vi "Read Assert.vi"(7 "Assert Only? (F)":bool, 8 "error in (no error)":errorcluster, 10 "VI Call Chain":string[](array[string]), 11 "Assert Factory in":refnum<class "Assert Factory.lvclass">) -> (0 "error out":errorcluster, 2 "Assert":refnum<class "Assert.lvclass">, 3 "Assert Factory out":refnum<class "Assert Factory.lvclass">)   [LabVIEW 2009, in "Caraya.lvlib" / "Assert Factory.lvclass"]
doc: "Returns the Assert implementation being used for a specific VI."
uses:
  Assert Factory.lvclass
  Assert/Assert.lvclass
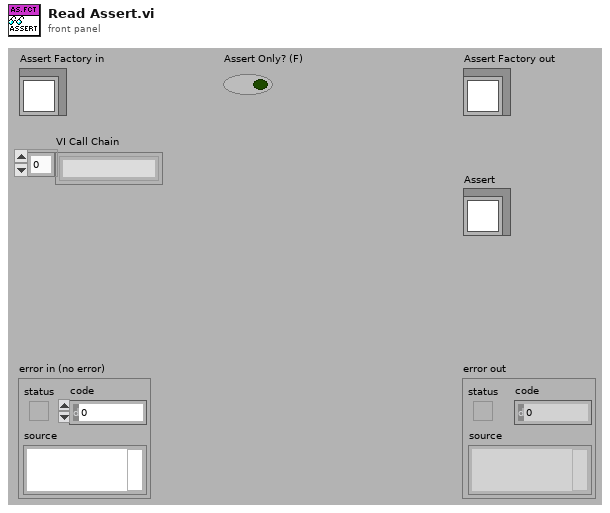
[diagram p1: front panel]
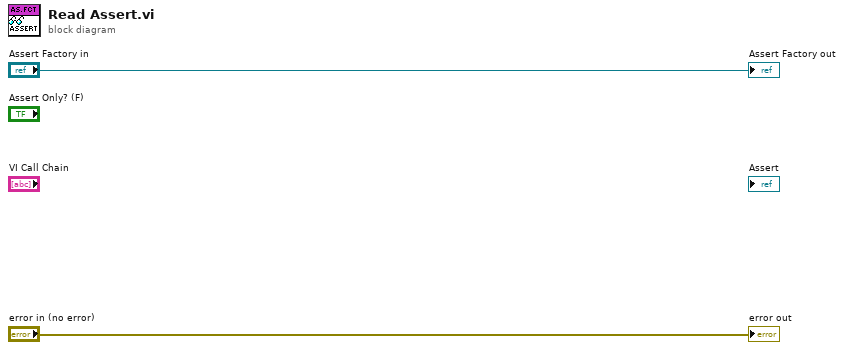
[diagram p0: block diagram]
diagram:
  "error out" <- "error in (no error)"
  "Assert Factory out" <- "Assert Factory in"
